vi "2_Trav_move_Checker.vi"(0 "Traverse Setups":string[](array[string]), 1 "Extra Command String":string, 3 "Home Z":T1, 5 "Traverse Positions (Tun Cord)":sgl[](array[numeric])=[0.0, 0.0, 0.0] format="%.2f", 7 "Display Error":bool=TRUE, 9 "Backlash Compensation?":bool=TRUE, 11 "Offset (Tun Cord) 1-2":sgl[](array[numeric]), 12 "Row Number":i32=11, 13 "Currently on Point":i32=11, 14 "Last Part of Move?":bool=TRUE) -> (4 "Trav Position achieved":sgl[](array[numeric]) format="%.2f", 6 "Error from Traverse named":string, 8 "Steps  for First Trav":sgl[][](array[numeric]) format="%#.0f", 15 "Error String":string)   [LabVIEW 2022 SP3]
uses:
  Controls/Home.ctl
  Trav_mode.ctl
  Controls/User_Specific_mode.ctl
  Controls/Tunnel_Coordinates.ctl
  Globals/Constants_global.vi
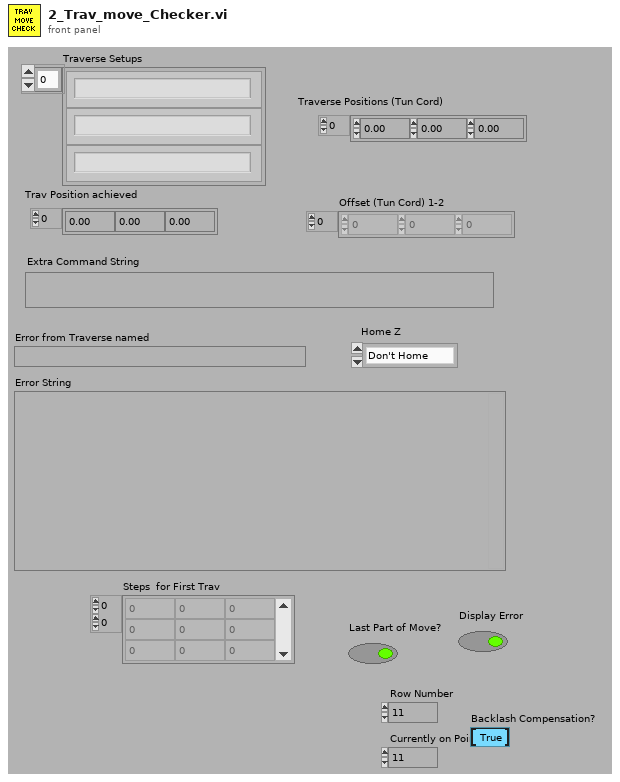
[diagram p1: front panel]
types:
  T1 = typedef "Home.ctl" = enum16{"Don't Home", "Home  +X", "Home  -X", "Home  +Y", "Home  -Y", "Home  +Z", "Home  -Z"}
  T2 = typedef "Tunnel_Coordinates.ctl" = enum16{"Work in Tunnel Coordinates", "Work in Model Coordinates"}
  T3 = typedef "User_Specific_mode.ctl" = enum16{"Check VI only", "Run VI"}
  T4 = typedef "Trav_mode.ctl" = enum16{"Move traverse", "Read traverse position", "Teach Position"}
  T5 = cluster{"Index":i32, "Move Steps (Tun Cord)":sgl[][]}
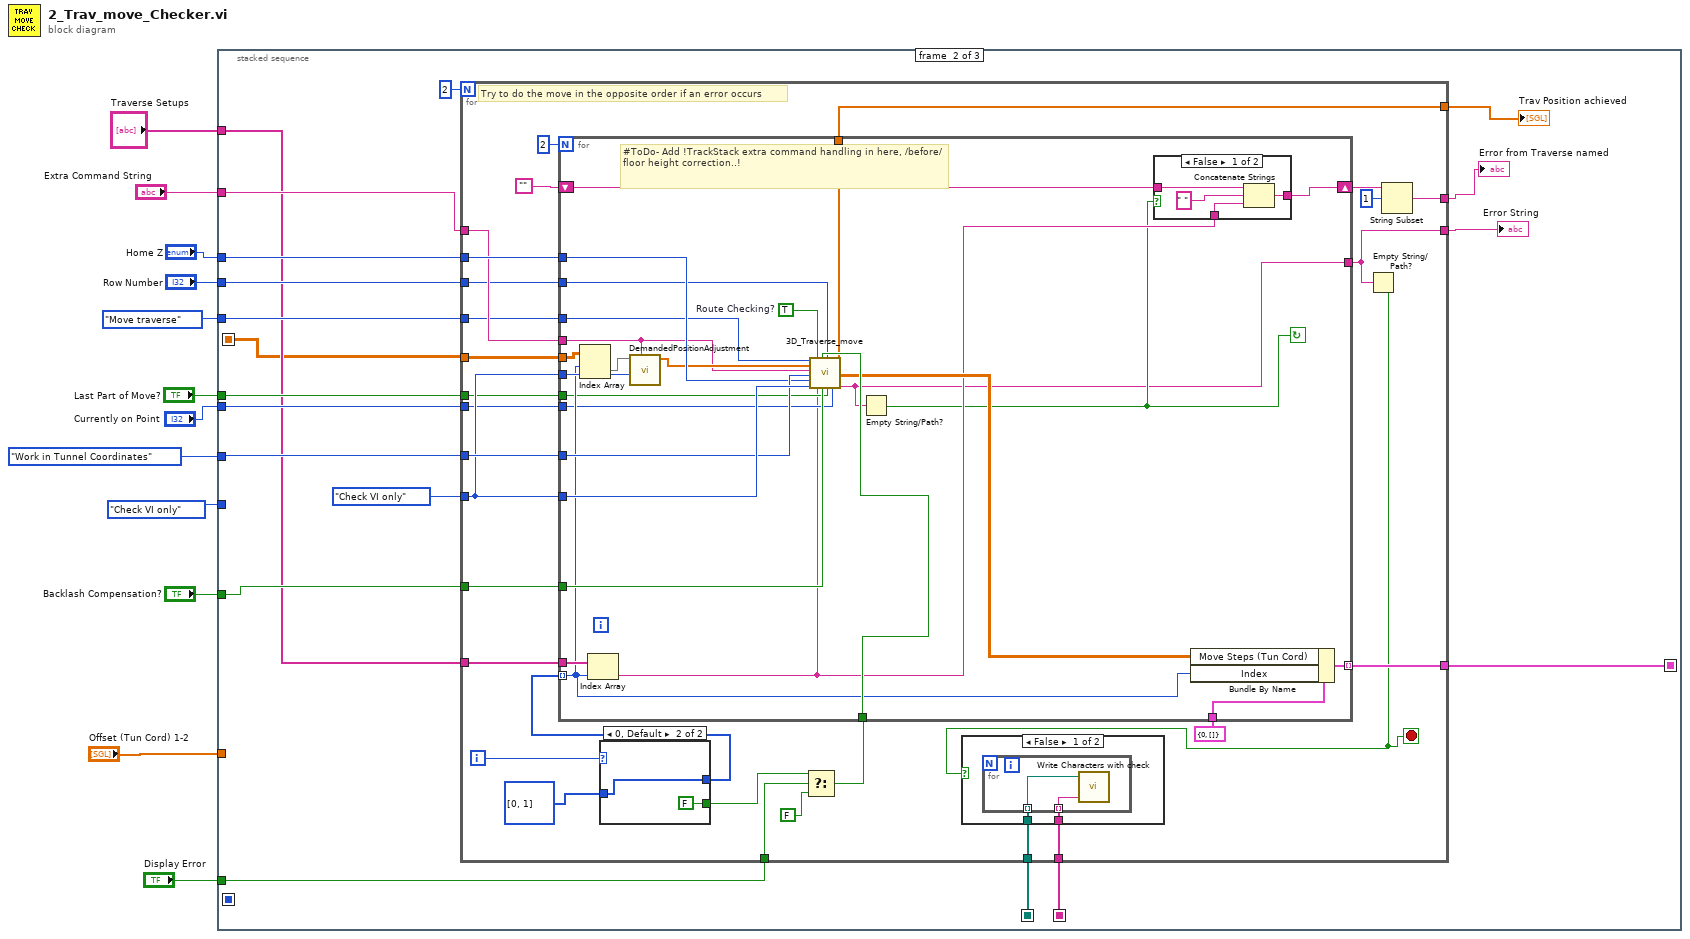
[diagram p0: block diagram]
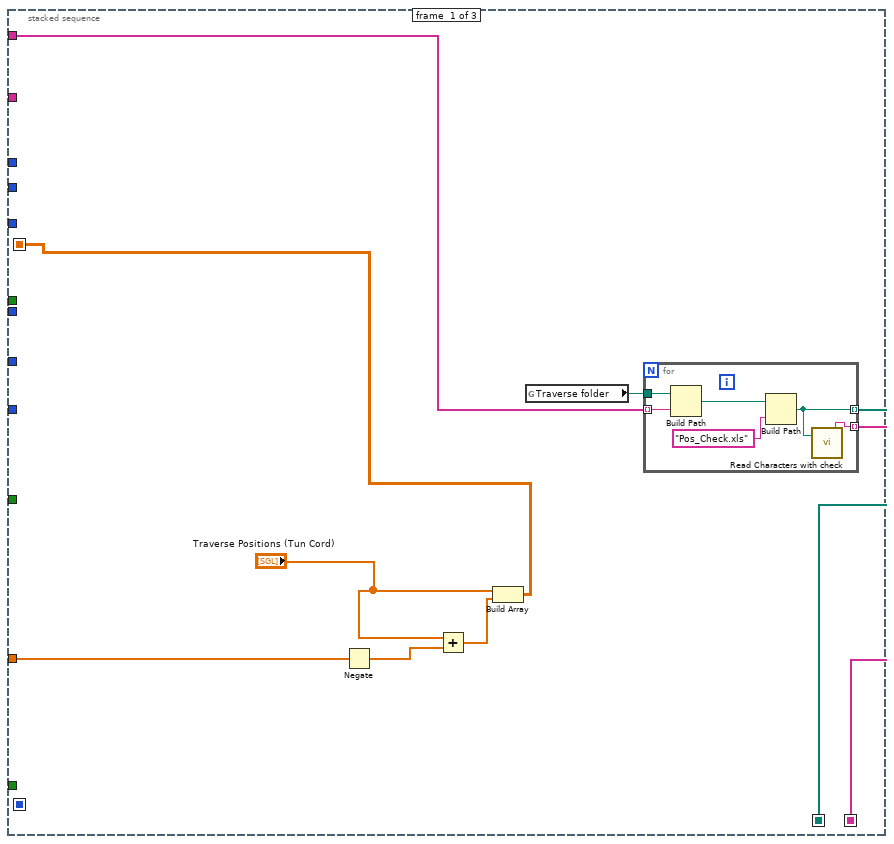
[diagram p2: hidden frame]
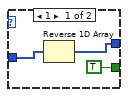
[diagram p4: hidden frame]
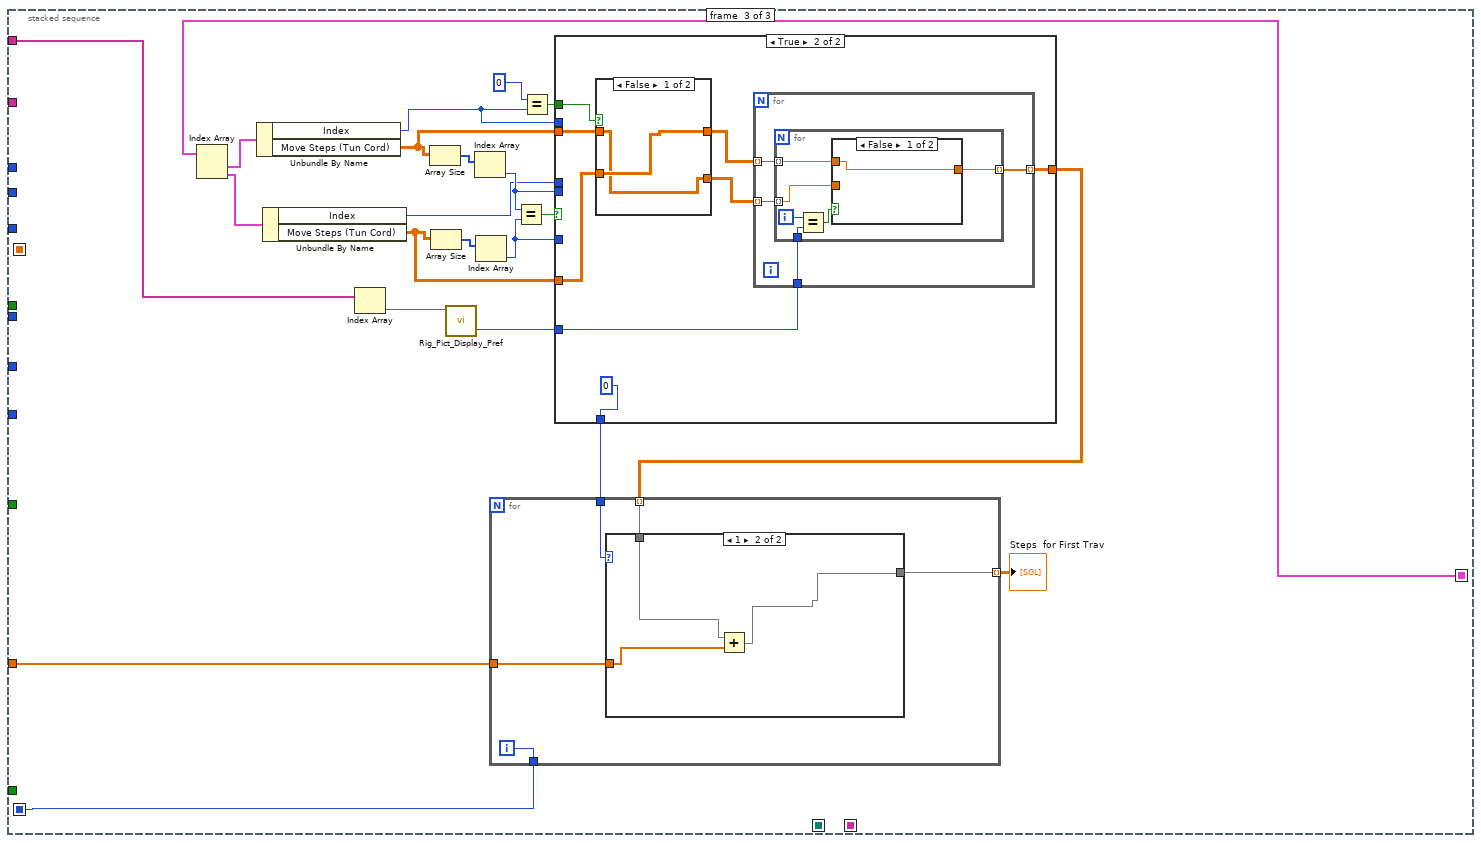
[diagram p6: hidden frame]
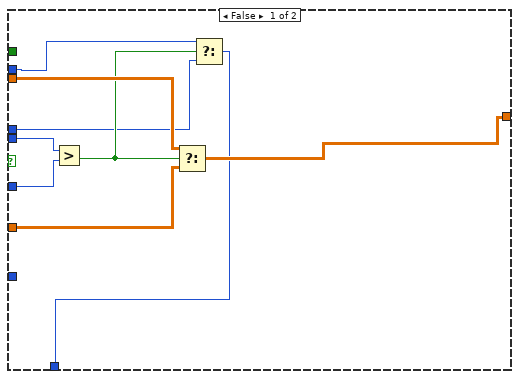
[diagram p8: hidden frame]
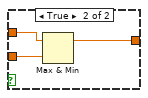
[diagram p9: hidden frame]
diagram:
  n1 = stacked-sequence {
    seq-local: [_ w42 _] -> [_ _ w126]
    seq-local: [w21 _ _] -> [_ w41 _]
    seq-local: [w20 _ _] -> [_ w40 _]
    seq-local: [_ _ w119] -> [_ _ _]
    seq-local: [w14 _ _] -> [_ w30 _]
    tunnel: "Extra Command String" -> [_ w46 _]
    tunnel: Tunnel_Coordinates."Work in Tunnel Coordinates" ("Work in Tunnel Coordinates?") -> [_ w44 _]
    tunnel: User_Specific_mode."Check VI only" ("Simulate/Run") -> [_ _ _]
    tunnel: "Backlash Compensation?" -> [_ w43 _]
    tunnel: "Display Error" -> [_ w28 _]
    tunnel: "Row Number" -> [_ w39 _]
    tunnel: Trav_mode."Move traverse" ("Mode") -> [_ w38 _]
    tunnel: "Last Part of Move?" -> [_ w37 _]
    tunnel: "Currently on Point" -> [_ w36 _]
    tunnel: "Home Z" -> [_ w35 _]
    tunnel: "Traverse Setups" -> [w18 w31 w118]
    tunnel: "Offset (Tun Cord) 1-2" -> [w13 _ w117]
    frame #0 {
      n2 = Negate(x=w13) -> (-x=w16:sgl[])
      n3 = Add(x="Traverse Positions (Tun Cord)", y=w16) -> (x+y=w17:sgl[])
      n4 = Build Array("Traverse Positions (Tun Cord)", w17) -> (w14:sgl[][])
      n5 = global read "Constants_global.vi" "Traverse folder"() -> (w19:path)
      n6 = for {
        tunnel: w19 -> [w25]
        tunnel: w18 -> [w24] mode=indexing
        tunnel: [w22] -> w21 mode=indexing
        tunnel: [w23] -> w20 mode=indexing
        n7 = Build Path(base path=w25, name or relative path=w24) -> (appended path=w26:path)
        n8 = Build Path(base path=w26, name or relative path="Pos_Check.xls" ("string")) -> (appended path=w23:path)
        n9 = call "Read Characters with check.vi"("file (use dialog)"=w23) -> ("Read String"=w22:string)  [unwired: 1 in, 1 out]
      }
    }
    frame #1 {
      n10 = for {
        N: 2 -> [_]
        tunnel: w43 -> [w76]
        tunnel: w44 -> [w75]
        tunnel: [w71] -> w33
        tunnel: w35 -> [w70]
        tunnel: w30 -> [w68]
        tunnel: User_Specific_mode."Check VI only" ("Simulate/Run") -> [w67]
        tunnel: w31 -> [w66]
        tunnel: w46 -> [w69]
        tunnel: [w52] -> w29
        tunnel: [w62] -> w42
        tunnel: w41 -> [w61]
        tunnel: w40 -> [w60]
        tunnel: w39 -> [w58]
        tunnel: w38 -> [w57]
        tunnel: w37 -> [w56]
        tunnel: w36 -> [w55]
        tunnel: [w54] -> w32
        tunnel: w28 -> [w49]
        i -> [w65]
        stop <- w51 stop-if-true
        # "Try to do the move in the opposite order if an error occurs"
        n11 = case shown="0, Default" w65 {
          tunnel: [w82 w85] -> w59
          tunnel: i32[] [0, 1] -> [w83 w85]
          tunnel: [TRUE FALSE] -> w48
          frame 1 {
            n12 = Reverse 1D Array(array=w83) -> (reversed array=w82:i32[])
          }
          frame 0, Default {
          }
        }
        n13 = Select(t=w48, s=w49, f=FALSE) -> (s? t:f=w47:bool)
        n14 = for {
          N: 2 -> [_]
          tunnel: w66 -> [w99]
          tunnel: w76 -> [w111]
          tunnel: w67 -> [w109]
          tunnel: w75 -> [w108]
          shift-right: [w107] -> w73
          shift-left: "" -> [w106]
          tunnel: w70 -> [w105]
          tunnel: w69 -> [w102]
          tunnel: w68 -> [w101]
          tunnel: w67 -> [w103]
          tunnel: w59 -> [w96] mode=indexing
          tunnel: w47 -> [w98]
          tunnel: T5 {"Index"=0, "Move Steps (Tun Cord)"=[]} -> [w97]
          tunnel: [w95] -> w62 mode=indexing
          tunnel: w58 -> [w94]
          tunnel: w57 -> [w93]
          tunnel: w56 -> [w92]
          tunnel: w55 -> [w91]
          tunnel: [w90] -> w54
          tunnel: [w86] -> w52
          stop <- w87 continue-if-true
          w110 = TRUE  # Route Checking?
          # "#ToDo- Add !TrackStack extra command handling in here, /before/ floor height correction..!"
          n15 = Index Array(array=w101, index (row)=w96) -> (element=w100:sgl[])  [unwired: 1 in]
          n16 = Index Array(array=w99, index=w96) -> (element=w88:string)
          n17 = call "DemandedPositionAdjustment.vi"("Extra Command String"=w102, "Simulate/Run"=w103, "Demanded Position"=w100) -> ("Adjusted Position"=w104:sgl[])  [unwired: 8 in]
          n18 = call "3D_Traverse_move.vi"("Mode"=w93, "Position"=w104, "Extra command String"=w102, "Work in Tunnel Coordinates"=w108, "Home"=w105, "Simulate/Run"=w109, "Route Checking?"=w110, "Traverse name"=w88, "Display Error"=w98, "Backlash Compensation?"=w111, "Row Number"=w94, "Last Part of Move?"=w92, "Currently on Point"=w91) -> ("Trav Position achieved"=w90:sgl[], "Valid Steps before Trav to Trav (Tun Cord)"=w89:sgl[][], "Error String"=w86:string)  [unwired: 3 in, 1 out]
          n19 = Empty String/Path?(string/path=w86) -> (empty?=w87:bool)
          n20 = case shown="False" w87 {
            tunnel: [w115 w116] -> w107
            tunnel: w106 -> [w114 w116]
            tunnel: w88 -> [w113 _]
            frame False {
              n21 = Concatenate Strings(w114, " " ("string"), w113) -> (w115:string)
            }
            frame True {
            }
          }
          n22 = Bundle By Name(cluster=w97, "Move Steps (Tun Cord)"=w89, "Index"=w96) -> (w95:T5)
        }
        n23 = Empty String/Path?(string/path=w52) -> (empty?=w51:bool)
        n24 = case shown="False" w51 {
          tunnel: w61 -> [w78 _]
          tunnel: w60 -> [w77 _]
          frame False {
            n25 = for {
              tunnel: w78 -> [w79] mode=indexing
              tunnel: w77 -> [w80] mode=indexing
              n26 = call "Write Characters with check.vi"("String to Write"=w79, "file (use dialog)"=w80) -> ()  [unwired: 2 in, 1 out]
            }
          }
          frame True {
          }
        }
        n27 = String Subset(string=w73, offset (0)=1) -> (substring=w71:string)  [unwired: 1 in]
      }
      "Error from Traverse named" <- w33
      "Trav Position achieved" <- w32
      "Error String" <- w29
    }
    frame #2 {
      n28 = Index Array(array=w126) -> (element #1=w128:T5, element #2=w129:T5)  [unwired: 2 in]
      n29 = Unbundle By Name(w128) -> ("Index"=w124:i32, "Move Steps (Tun Cord)"=w134:sgl[][])
      n30 = Unbundle By Name(w129) -> ("Index"=w123:i32, "Move Steps (Tun Cord)"=w135:sgl[][])
      n31 = Index Array(array=w118) -> (element=w125:string)  [unwired: 1 in]
      n32 = Array Size(array=w134) -> (size(s)=w130:i32[])
      n33 = Array Size(array=w135) -> (size(s)=w131:i32[])
      n34 = call "Rig_Pict_Display_Pref.vi"("Traverse Name"=w125) -> ("Which Axis is vertical?"=w136:enum16{"X Axis", "Y Axis", "Z Axis"})  [unwired: 7 out]
      n35 = Index Array(array=w130) -> (element=w137:i32)  [unwired: 1 in]
      n36 = Index Array(array=w131) -> (element=w138:i32)  [unwired: 1 in]
      n37 = Equal?(x=w137, y=w138) -> (x = y?=w132:bool)
      n38 = Equal?(x=0, y=w124) -> (x = y?=w133:bool)
      n39 = case shown="True" w132 {
        tunnel: w133 -> [_ w164]
        tunnel: w134 -> [w154 w163]
        tunnel: w135 -> [w153 w160]
        tunnel: w136 -> [_ w159]
        tunnel: w137 -> [w156 _]
        tunnel: w138 -> [w155 _]
        tunnel: [w152 w158] -> w122
        tunnel: w124 -> [w150 _]
        tunnel: w123 -> [w149 _]
        tunnel: [w148 0 ("x")] -> w121
        frame False {
          n40 = Greater?(x=w156, y=w155) -> (0:w151:bool)
          n41 = Select(t=w154, s=w151, f=w153) -> (s? t:f=w152:sgl[][])
          n42 = Select(t=w150, s=w151, f=w149) -> (s? t:f=w148:i32)
        }
        frame True {
          n43 = case shown="False" w164 {
            tunnel: [w180 w182] -> w162
            tunnel: w163 -> [w179 w182]
            tunnel: [w179 w181] -> w161
            tunnel: w160 -> [w180 w181]
            frame False {
            }
            frame True {
            }
          }
          n44 = for {
            tunnel: w162 -> [w168] mode=indexing
            tunnel: w161 -> [w167] mode=indexing
            tunnel: w159 -> [w166]
            tunnel: [w165] -> w158 mode=indexing
            n45 = for {
              tunnel: w168 -> [w171] mode=indexing
              tunnel: w167 -> [w170] mode=indexing
              tunnel: w166 -> [w173]
              tunnel: [w169] -> w165 mode=indexing
              i -> [w174]
              n46 = Equal?(x=w174, y=w173) -> (x = y?=w172:bool)
              n47 = case shown="False" w172 {
                tunnel: w171 -> [w175 w178]
                tunnel: w170 -> [_ w177]
                tunnel: [w175 w176] -> w169
                frame False {
                }
                frame True {
                  n48 = Max & Min(x=w178, y=w177) -> (max(x,y)=w176:sgl)  [unwired: 1 out]
                }
              }
            }
          }
        }
      }
      n49 = for {
        tunnel: w122 -> [w142] mode=indexing
        tunnel: w121 -> [w143]
        tunnel: w117 -> [w141]
        tunnel: [w140] -> w120 mode=indexing
        tunnel: [w139] -> w119
        i -> [w139]
        n50 = case shown="1" w143 {
          tunnel: w142 -> [w144 w146]
          tunnel: w141 -> [_ w147]
          tunnel: [w144 w145] -> w140
          frame 0, Default {
          }
          frame 1 {
            n51 = Add(x=w146, y=w147) -> (x+y=w145:sgl[])
          }
        }
      }
      "Steps  for First Trav" <- w120
    }
  }
